vi "Split Digits.vi"(0 "Input":u16) -> (1 "Digit 4":u16, 2 "Digit 3":u16, 3 "Digit 2":u16, 4 "Digit 1":u16)   [LabVIEW 2015]
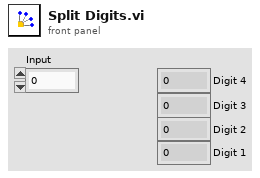
[diagram p1: front panel]
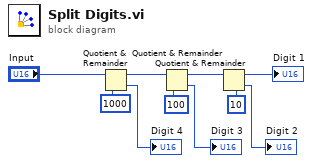
[diagram p0: block diagram]
diagram:
  n1 = Quotient & Remainder(x="Input", y=u16 1000) -> (x-y*floor(x/y)=w7:u16, floor(x/y)=→"Digit 4":u16)
  n2 = Quotient & Remainder(x=w7, y=u16 100) -> (x-y*floor(x/y)=w3:u16, floor(x/y)=→"Digit 3":u16)
  n3 = Quotient & Remainder(x=w3, y=u16 10) -> (x-y*floor(x/y)=→"Digit 1":u16, floor(x/y)=→"Digit 2":u16)
